vi "read_In.vi"() -> (0 "INMFC1":dbl, 1 "Remote":bool, 2 "Run":bool, 3 "Bubbler In":bool, 4 "Active":bool)   [LabVIEW 2011]
uses:
  low_level_proc/globals.vi
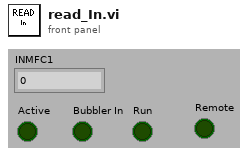
[diagram p1: front panel]
types:
  T1 = typedef "relaySpec.ctl" = cluster{"Card Index":u16, "Relay Index":u16}
  T2 = typedef "DA_Spec.ctl" = cluster{"Card Index":u16, "Channel Index":u16}
  T3 = typedef "AD_Spec.ctl" = u16
  T4 = cluster{"Relay Functions":cluster{"Remote":T1, "Active":T1, "Bubbler In":T1, "Run":T1}, "D/A Functions":cluster{"Flow":T2}, "Flow Ranges":cluster{"Flow (INMFC1)":u16}, "A/D Functions":cluster{"Flow":T3}}
  T5 = cluster{"Remote":T1, "Active":T1, "Bubbler In":T1, "Run":T1}
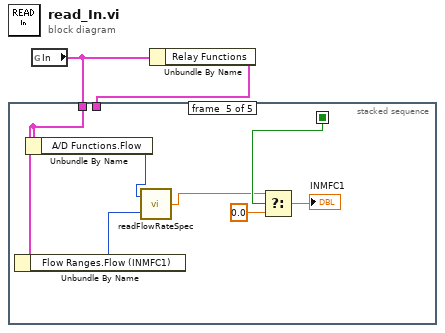
[diagram p0: block diagram]
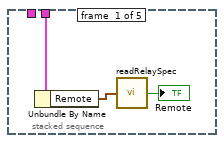
[diagram p2: hidden frame]
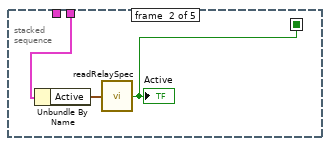
[diagram p3: hidden frame]
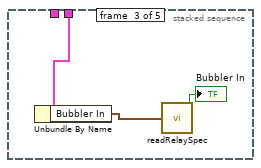
[diagram p4: hidden frame]
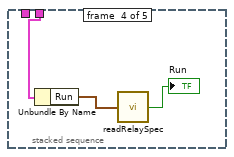
[diagram p5: hidden frame]
diagram:
  n1 = global read "globals.vi" "In"() -> (w1:T4)
  n2 = Unbundle By Name(w1) -> ("Relay Functions"=w2:T5)
  n3 = stacked-sequence {
    seq-local: [_ w8 _ _ _] -> [_ _ _ _ w21]
    tunnel: w2 -> [w4 w6 w10 w13 _]
    tunnel: w1 -> [_ _ _ _ w18]
    frame #0 {
      n4 = Unbundle By Name(w4) -> ("Remote"=w3:T1)
      n5 = call "readRelaySpec.vi"("RelaySpec"=w3) -> ("Relay Status"=→"Remote":bool)
    }
    frame #1 {
      n6 = Unbundle By Name(w6) -> ("Active"=w7:T1)
      n7 = call "readRelaySpec.vi"("RelaySpec"=w7) -> ("Relay Status"=w8:bool)
      "Active" <- w8
    }
    frame #2 {
      n8 = Unbundle By Name(w10) -> ("Bubbler In"=w9:T1)
      n9 = call "readRelaySpec.vi"("RelaySpec"=w9) -> ("Relay Status"=→"Bubbler In":bool)
    }
    frame #3 {
      n10 = Unbundle By Name(w13) -> ("Run"=w12:T1)
      n11 = call "readRelaySpec.vi"("RelaySpec"=w12) -> ("Relay Status"=→"Run":bool)
    }
    frame #4 {
      n12 = Unbundle By Name(w18) -> ("Flow Ranges.Flow (INMFC1)"=w16:u16)
      n13 = Unbundle By Name(w18) -> ("A/D Functions.Flow"=w17:T3)
      n14 = call "readFlowRateSpec.vi"("Flow range Index"=w16, "Channel Index"=w17) -> ("Flow Rate (sccm)"=w15:dbl)
      n15 = Select(t=w15, s=w21, f=0.0) -> (s? t:f=→"INMFC1":dbl)
    }
  }
